vi "Teleop.vi"(10 "Match Info":T1={"Autonomous Elapsed Seconds"=0.0, "TeleOp Elapsed Seconds"=0.0, "Disabled Elapsed Seconds"=0.0, "Visited Autonomous"=FALSE, "Visited TeleOp"=FALSE, "Visited Disabled"=FALSE, "Autonomous Settings"={"Autonomous Style"=enum."Independent", "VI Refnum"=refnum}}, 11 "Call Context":T2) -> ()   [LabVIEW 2015]
doc: "This VI is called for each TeleOp packet received from the DS where the robot is not disabled. It is often used to read from the joysticks and update I/O or to update setpoints for timed control loops. It should complete and return within 20 milliseconds or it may miss DS packets."
uses:
  <vilib>/Rock Robotics/WPI/DriverStation/WPI_DriverStationDerivedRobotMode.ctl
  <vilib>/Rock Robotics/WPI/DriverStation/WPI_DriverStationMatch Info.ctl
  <vilib>/Rock Robotics/WPI/Utilities/WPI_GetSetVariantRefNum.vi
  <vilib>/Rock Robotics/Network Tables/NT Write Boolean Array.vi
  <vilib>/Rock Robotics/Network Tables/NT Write Numeric Array.vi
  <vilib>/Rock Robotics/Network Tables/NT Read Boolean.vi
  <vilib>/Rock Robotics/Network Tables/NT Read Number.vi
panel:
  out "Sample Slider 0":dbl(slide) scale=0.0..5.0
  out "Sample Boolean 1":bool
  out "Sample Boolean 0":bool
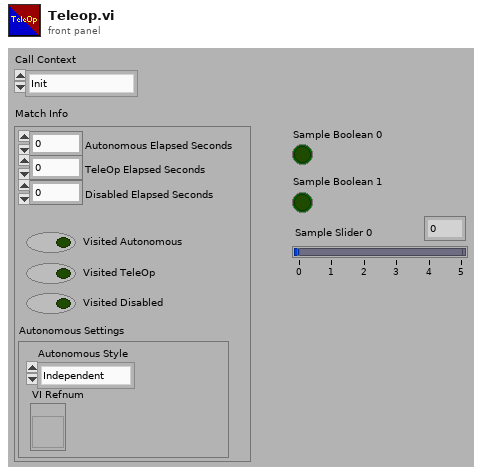
[diagram p1: front panel]
types:
  T1 = typedef "WPI_DriverStationMatch Info.ctl" = cluster{"Autonomous Elapsed Seconds":dbl, "TeleOp Elapsed Seconds":dbl, "Disabled Elapsed Seconds":dbl, "Visited Autonomous":bool, "Visited TeleOp":bool, "Visited Disabled":bool, "Autonomous Settings":cluster{"Autonomous Style":enum16{"Iterative", "Independent"}, "VI Refnum":refnum<vi>}}
  T2 = typedef "WPI_DriverStationDerivedRobotMode.ctl" = enum16{"Init", "Execute", "Stop"}
  T3 = typedef "WPI_JoystickDevRef.ctl" = cluster{"Device":T4}
  T4 = typedef "WPI_JoystickDeviceEnum.ctl" = enum16{"USB 0", "USB 1", "USB 2", "USB 3", "USB 4", "USB 5"}
  T5 = cluster{"Axes[0]":dbl, "Axes[1]":dbl, "Axes[2]":dbl, "Axes[3]":dbl, "Axes[4]":dbl, "Axes[5]":dbl, "Axes[6]":dbl, "Axes[7]":dbl, "Axes[8]":dbl}
  T6 = typedef "WPI_MotorControlDeviceRef.ctl" = cluster{"DeviceStatus":errorcluster, "Type":T7, "PWM":cluster{"PWM Channel":T8, "DeadBand":T9}, "CAN":cluster{"Device Number":u8, "Control Mode":T10, "Semaphore":T11, "Max Vout":dbl, "TalonSRX Control Mode":T12}, "Invert":bool}
  T7 = typedef "WPI_MotorControlType.ctl" = enum16{"PWM", "CAN", "CANTalonSRX"}
  T8 = typedef "FPGA_DIOPWMChannel.ctl" = enum8{"PWM 0", "PWM 1", "PWM 2", "PWM 3", "PWM 4", "PWM 5", "PWM 6", "PWM 7", "PWM 8", "PWM 9", "PWM MXP 0", "PWM MXP 1", "PWM MXP 2", "PWM MXP 3", "PWM MXP 4", "PWM MXP 5", "PWM MXP 6", "PWM MXP 7", "PWM MXP 8", "PWM MXP 9", "Invalid"}
  T9 = typedef "WPI_PWMDeadband.ctl" = cluster{"Name":string, "maxPositivePwm":i32, "minPositivePwm":i32, "centerPwm":i32, "maxNegativePwm":i32, "minNegativePwm":i32, "angularRange":u16}
  T10 = typedef "WPI_CANJaguar_ControlMode.ctl" = enum8{"Percent VBus", "Current", "Speed", "Position", "Voltage"}
  T11 = typedef "Semaphore RefNum" = refnum<k1>
  T12 = typedef "WPI_CANTalonSRX_APIControlMode.ctl" = enum8{"Percent VBus", "Speed", "Position", "Slave", "Unchanged / Invalid", "Voltage Compensation", "Current", "Motion Profile"}
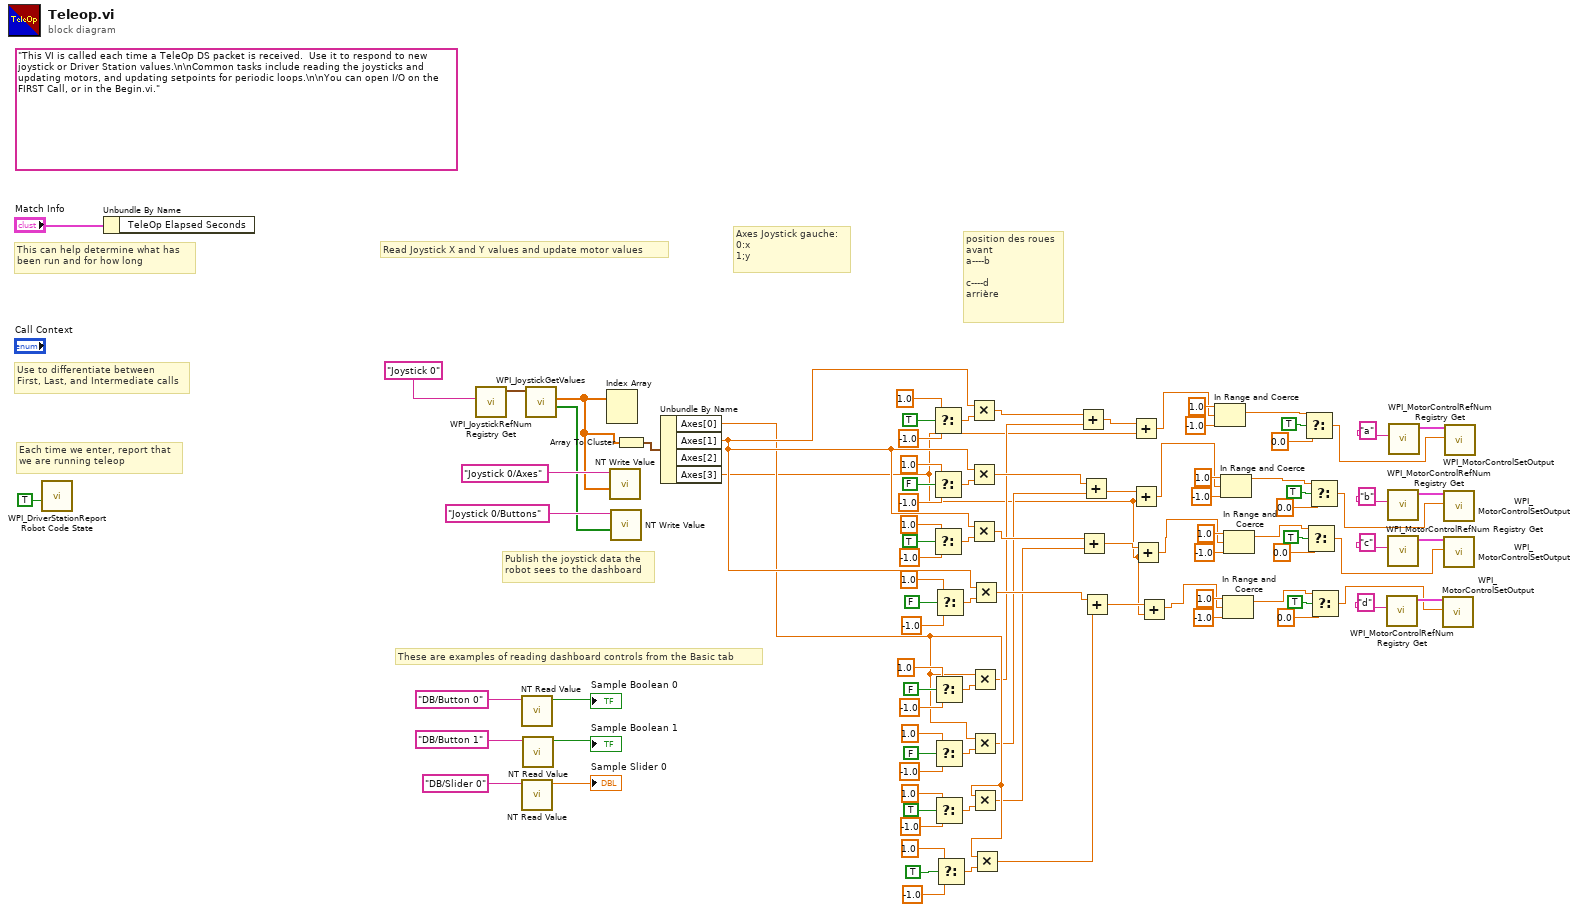
[diagram p0: block diagram]
diagram:
  (unwired) "This VI is called each time a TeleOp DS packet is received.  Use it to respond to new joystick or Driver Station values.\n\nCommon tasks include reading the joysticks and updating motors, and updating setpoints for periodic loops.\n\nYou can open I/O on the FIRST Call, or in the Begin.vi."
  # "position des roues\navant\na----b\n\nc----d\narrière"
  # "Axes Joystick gauche:\n0:x\n1;y"
  # "These are examples of reading dashboard controls from the Basic tab"
  # "Publish the joystick data the\nrobot sees to the dashboard"
  # "Each time we enter, report that\nwe are running teleop"
  # "Use to differentiate between\nFirst, Last, and Intermediate calls"
  # "This can help determine what has\nbeen run and for how long"
  # "Read Joystick X and Y values and update motor values"
  n1 = call <vilib>:"WPI_DriverStationReport Robot Code State.vi"("TeleOp"=TRUE ("Autonomous")) -> ()  [unwired: 10 in, 1 out]
  n2 = Unbundle By Name("Match Info") -> ()  [unwired: 1 out]
  n3 = call <vilib>:"WPI_JoystickRefNum Registry Get.vi"("refnum name"="Joystick 0") -> ("JoystickDevRef"=w96:T3)  [unwired: 1 in, 9 out]
  n4 = call-poly <vilib>:"NT Read Value.vi"("Name"="DB/Button 0" ("refnum name")) -> ("Boolean"=→"Sample Boolean 0":bool)  [unwired: 9 in, 1 out]
  n5 = call-poly <vilib>:"NT Read Value.vi"("Name"="DB/Slider 0" ("refnum name")) -> ("Numeric"=→"Sample Slider 0":dbl)  [unwired: 9 in, 1 out]
  n6 = call-poly <vilib>:"NT Read Value.vi"("Name"="DB/Button 1" ("refnum name")) -> ("Boolean"=→"Sample Boolean 1":bool)  [unwired: 9 in, 1 out]
  n7 = call <vilib>:"WPI_JoystickGetValues.vi"("JoystickDevRef"=w96) -> ("Buttons"=w92:bool[], "Axes"=w85:dbl[])  [unwired: 6 in, 3 out]
  n8 = Index Array(array=w85) -> ()  [unwired: 2 in, 2 out]
  n9 = call-poly <vilib>:"NT Write Value.vi"("Numeric Array"=w85, "Name"="Joystick 0/Axes") -> ()  [unwired: 9 in, 1 out]
  n10 = call-poly <vilib>:"NT Write Value.vi"("Boolean Array"=w92, "Name"="Joystick 0/Buttons") -> ()  [unwired: 9 in, 1 out]
  n11 = Array To Cluster(array=w85) -> (cluster=w84:T5)
  n12 = Unbundle By Name(w84) -> ("Axes[0]"=w34:dbl, "Axes[1]"=w51:dbl, "Axes[3]"=w6:dbl)  [unwired: 1 out]
  n13 = Select(t=1.0, s=TRUE, f=-1.0) -> (s? t:f=w72:dbl)
  n14 = Select(t=1.0, s=FALSE, f=-1.0) -> (s? t:f=w71:dbl)
  n15 = Select(t=1.0, s=TRUE, f=-1.0) -> (s? t:f=w64:dbl)
  n16 = Select(t=1.0, s=FALSE, f=-1.0) -> (s? t:f=w38:dbl)
  n17 = Select(t=1.0, s=FALSE, f=-1.0) -> (s? t:f=w39:dbl)
  n18 = Select(t=1.0, s=TRUE, f=-1.0) -> (s? t:f=w46:dbl)
  n19 = Select(t=1.0, s=FALSE, f=-1.0) -> (s? t:f=w63:dbl)
  n20 = Select(t=1.0, s=TRUE, f=-1.0) -> (s? t:f=w47:dbl)
  n21 = Multiply(x=w51, y=w72) -> (x*y=w33:dbl)
  n22 = Multiply(x=w51, y=w71) -> (x*y=w32:dbl)
  n23 = Multiply(x=w51, y=w64) -> (x*y=w31:dbl)
  n24 = Multiply(x=w34, y=w38) -> (x*y=w26:dbl)
  n25 = Multiply(x=w34, y=w39) -> (x*y=w27:dbl)
  n26 = Multiply(x=w34, y=w46) -> (x*y=w28:dbl)
  n27 = Multiply(x=w51, y=w63) -> (x*y=w30:dbl)
  n28 = Multiply(x=w34, y=w47) -> (x*y=w29:dbl)
  n29 = Add(x=w33, y=w26) -> (x+y=w10:dbl)
  n30 = Add(x=w31, y=w28) -> (x+y=w8:dbl)
  n31 = Add(x=w32, y=w27) -> (x+y=w9:dbl)
  n32 = Add(x=w30, y=w29) -> (x+y=w7:dbl)
  n33 = Add(x=w10, y=w6) -> (x+y=w5:dbl)
  n34 = Add(x=w9, y=w6) -> (x+y=w4:dbl)
  n35 = Add(x=w8, y=w6) -> (x+y=w3:dbl)
  n36 = Add(x=w7, y=w6) -> (x+y=w1:dbl)
  n37 = In Range and Coerce(upper limit=1.0, x=w5, lower limit=-1.0) -> (coerced(x)=w18:dbl)  [unwired: 1 out]
  n38 = In Range and Coerce(upper limit=1.0, x=w4, lower limit=-1.0) -> (coerced(x)=w17:dbl)  [unwired: 1 out]
  n39 = In Range and Coerce(upper limit=1.0, x=w1, lower limit=-1.0) -> (coerced(x)=w15:dbl)  [unwired: 1 out]
  n40 = In Range and Coerce(upper limit=1.0, x=w3, lower limit=-1.0) -> (coerced(x)=w16:dbl)  [unwired: 1 out]
  n41 = Select(t=w18, s=TRUE, f=0.0) -> (s? t:f=w52:dbl)
  n42 = Select(t=w16, s=TRUE, f=0.0) -> (s? t:f=w54:dbl)
  n43 = Select(t=w17, s=TRUE, f=0.0) -> (s? t:f=w53:dbl)
  n44 = Select(t=w15, s=TRUE, f=0.0) -> (s? t:f=w55:dbl)
  n45 = call <vilib>:"WPI_MotorControlRefNum Registry Get.vi"("refnum name"="d") -> ("MotorControlDevRef"=w77:T6)  [unwired: 9 in, 1 out]
  n46 = call <vilib>:"WPI_MotorControlRefNum Registry Get.vi"("refnum name"="b") -> ("MotorControlDevRef"=w81:T6)  [unwired: 9 in, 1 out]
  n47 = call <vilib>:"WPI_MotorControlRefNum Registry Get.vi"("refnum name"="c") -> ("MotorControlDevRef"=w78:T6)  [unwired: 9 in, 1 out]
  n48 = call <vilib>:"WPI_MotorControlRefNum Registry Get.vi"("refnum name"="a") -> ("MotorControlDevRef"=w82:T6)  [unwired: 9 in, 1 out]
  n49 = call <vilib>:"WPI_MotorControlSetOutput.vi"("Output"=w55, "MotorControlDevRef"=w77) -> ()  [unwired: 7 in, 3 out]
  n50 = call <vilib>:"WPI_MotorControlSetOutput.vi"("Output"=w53, "MotorControlDevRef"=w81) -> ()  [unwired: 7 in, 3 out]
  n51 = call <vilib>:"WPI_MotorControlSetOutput.vi"("Output"=w54, "MotorControlDevRef"=w78) -> ()  [unwired: 7 in, 3 out]
  n52 = call <vilib>:"WPI_MotorControlSetOutput.vi"("Output"=w52, "MotorControlDevRef"=w82) -> ()  [unwired: 7 in, 3 out]
